vi "Discover Channels.vi"(8 "error in (no error)":errorcluster, 9 "module configurations":refnum<class "TBM module configuration.lvclass">[](array[class]), 10 "modules":refnum<class "TBM module execution interface.lvclass">[](array[class]), 11 "engine configuration":refnum<class "engine configuration.lvclass">) -> (0 "error out":errorcluster, 1 "module configurations out":refnum<class "TBM module configuration.lvclass">[](array[class]), 2 "modules out":refnum<class "TBM module execution interface.lvclass">[](array[class]), 3 "engine configuration out":refnum<class "engine configuration.lvclass">)   [LabVIEW 2014, in "Engine Runtime Interface.lvclass"]
doc: "This VI calls the 'Discover Channels' method for each module that was input and configured to enable this functionality. Channel discovery only occurrs if one or more modules are configured to map to channels dynamically."
uses:
  Engine Runtime Interface.lvclass
  <vilib>/NI/Tag Bus Module Framework/runtime/TBM module execution interface.lvclass
  <vilib>/NI/Tag Bus Module Framework/module configuration/TBM module configuration.lvclass
  Engine Configuration/engine configuration.lvclass
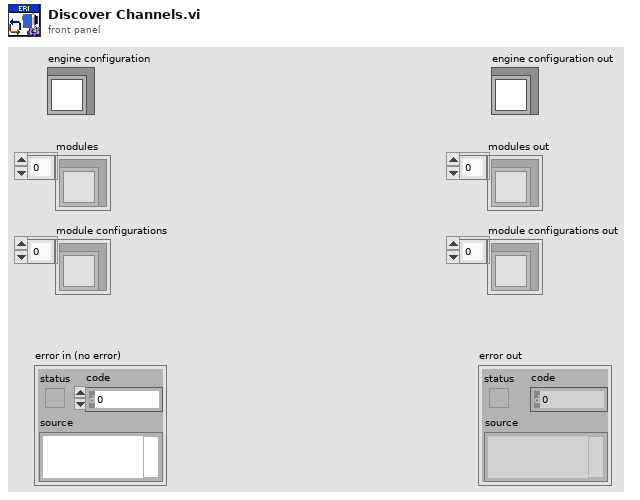
[diagram p1: front panel]
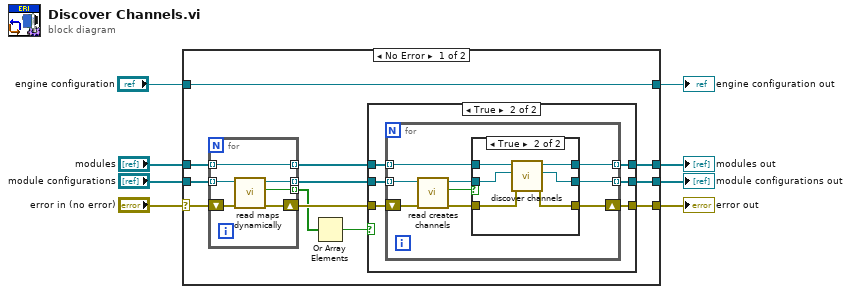
[diagram p0: block diagram]
diagram:
  n1 = case shown="No Error" "error in (no error)" {
    selector: "error in (no error)" -> [w12 w57]
    tunnel: [w19 w57] -> w7
    tunnel: [w20 w56] -> w2
    tunnel: "engine configuration" -> [w20 w56]
    tunnel: "modules" -> [w16 w54]
    tunnel: "module configurations" -> [w14 w55]
    tunnel: [w18 w54] -> w4
    tunnel: [w17 w55] -> w3
    frame No Error {
      n2 = for {
        tunnel: w16 -> [w53] mode=indexing
        tunnel: [w53] -> w15 mode=indexing
        tunnel: w14 -> [w52] mode=indexing
        tunnel: [w51] -> w13 mode=indexing
        shift-right: [w49] -> w11
        shift-left: w12 -> [w50]
        tunnel: [w48] -> w10 mode=indexing
        n3 = call-dynamic "read maps dynamically.vi"("error in"=w50, "module configuration in"=w52) -> ("error out"=w49:errorcluster, "maps dynamically"=w48:bool, "module configuration out"=w51:refnum<class "TBM module configuration.lvclass">)  [unwired: 7 in]
      }
      n4 = Or Array Elements(Boolean array=w10) -> (logical OR=w9:bool)
      n5 = case shown="True" w9 {
        tunnel: [w21 w29] -> w19
        tunnel: [w23 w28] -> w18
        tunnel: [w22 w27] -> w17
        tunnel: w15 -> [w23 w26]
        tunnel: w13 -> [w22 w25]
        tunnel: w11 -> [w21 w24]
        frame False {
          # "Don't discover channels if no one will map to them."
        }
        frame True {
          n6 = for {
            tunnel: w26 -> [w35] mode=indexing
            tunnel: w25 -> [w34] mode=indexing
            shift-right: [w32] -> w29
            shift-left: w24 -> [w33]
            tunnel: [w31] -> w28 mode=indexing
            tunnel: [w30] -> w27 mode=indexing
            n7 = call-dynamic "read creates channels.vi"("error in"=w33, "module configuration in"=w34) -> ("error out"=w37:errorcluster, "creates channels?"=w36:bool, "module configuration out"=w38:refnum<class "TBM module configuration.lvclass">)  [unwired: 7 in]
            n8 = case shown="True" w36 {
              tunnel: w38 -> [w40 w47]
              tunnel: w35 -> [w41 w46]
              tunnel: [w41 w45] -> w31
              tunnel: [w40 w44] -> w30
              tunnel: [w39 w42] -> w32
              tunnel: w37 -> [w39 w43]
              frame False {
              }
              frame True {
                n9 = call-dynamic "discover channels.vi"("error in"=w43, "module configuration"=w47, "module in"=w46) -> ("error out"=w42:errorcluster, "updated configuration"=w44:refnum<class "TBM module configuration.lvclass">, "module out"=w45:refnum<class "TBM module execution interface.lvclass">)  [unwired: 6 in]
              }
            }
          }
        }
      }
    }
    frame Error {
    }
  }
  "error out" <- w7
  "module configurations out" <- w3
  "modules out" <- w4
  "engine configuration out" <- w2
